vi "Set Progress Window Iteration.vi"(5 "current iteration":i32, 7 "total iterations":i32, 8 "error in (no error)":errorcluster, 10 "Status Message":string, 11 "DVRs in":T1) -> (0 "error out":errorcluster, 3 "DVRs out":T1)   [LabVIEW 2019, in "Build Automation.lvlib"]
uses:
  Build Automation.lvlib
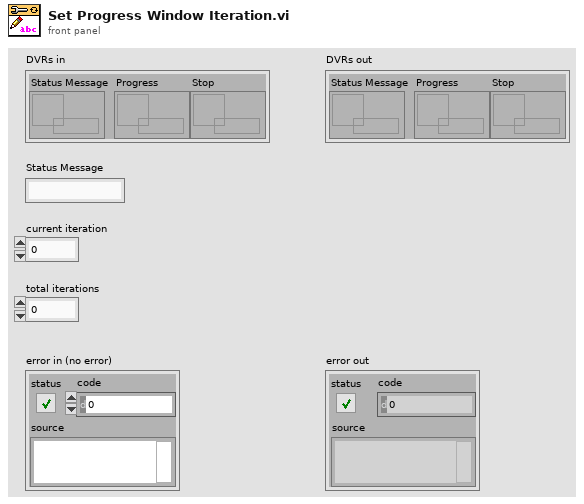
[diagram p1: front panel]
types:
  T1 = cluster{"Status Message":refnum<data-value>, "Progress":refnum<data-value>, "Stop":refnum<data-value>}
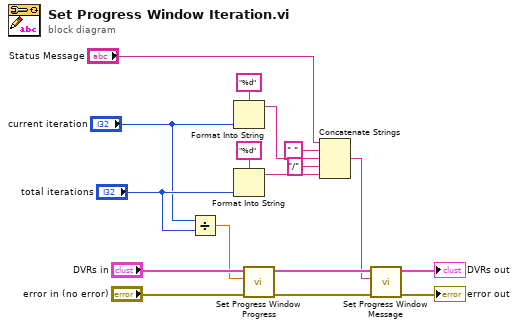
[diagram p0: block diagram]
diagram:
  n1 = Divide(x="current iteration", y="total iterations") -> (x/y=w3:dbl)
  n2 = Format Into String(format string="%d", "current iteration") -> (resulting string=w16:string)  [unwired: 2 in, 1 out]
  n3 = Format Into String(format string="%d", "total iterations") -> (resulting string=w13:string)  [unwired: 2 in, 1 out]
  n4 = call "Set Progress Window Progress.vi"("error in (no error)"="error in (no error)", "Progress"=w3, "DVRs in"="DVRs in") -> ("error out"=w6:errorcluster, "DVRs out"=w9:T1)  [unwired: 7 in]
  n5 = Concatenate Strings("Status Message", " " ("string"), w16, "/" ("string"), w13) -> (w8:string)
  n6 = call "Set Progress Window Message.vi"("error in (no error)"=w6, "Status Message"=w8, "DVRs in"=w9) -> ("error out"=→"error out":errorcluster, "DVRs out"=→"DVRs out":T1)  [unwired: 7 in]
